vi "Generate write queue item.vi"(8 "error in (no error)":errorcluster, 10 "Request ID":u64, 11 "ICallRequest":refnum<class "ICallRequest.lvclass">) -> (0 "error out":errorcluster, 3 "Write queue item":T1)   [LabVIEW 2020, in "wamplv.lvlib" / "ICallRequest.lvclass"]
uses:
  ICallRequest.lvclass
  WAMP Client/Private/TypeDef/Write queue item.ctl
  TypeDefs/Transport type.ctl
  wamplv.lvlib
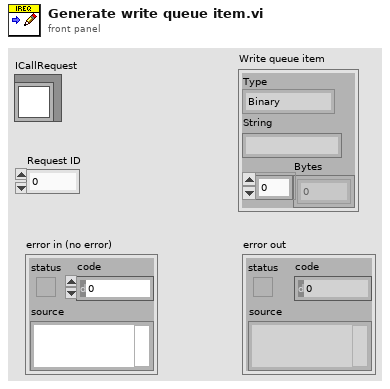
[diagram p1: front panel]
types:
  T1 = typedef "wamplv.lvlib/Write queue item.ctl" = cluster{"Type":T2, "String":string, "Bytes":u8[]}
  T2 = typedef "wamplv.lvlib/Transport type.ctl" = enum16{"Binary", "Text"}
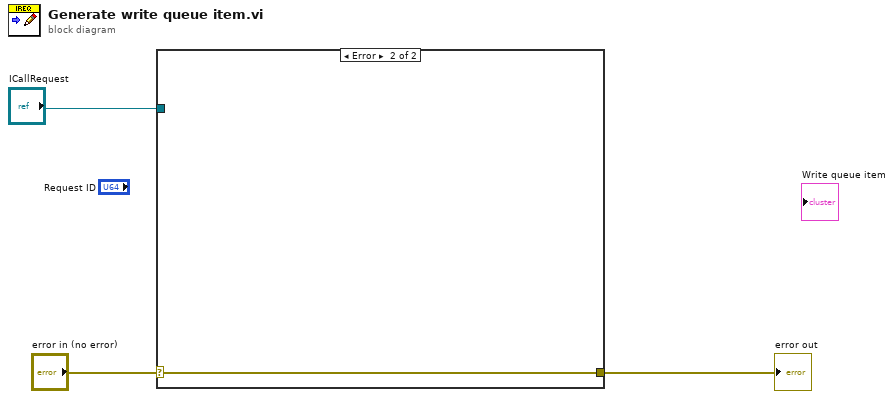
[diagram p0: block diagram]
diagram:
  n1 = case shown="Error" "error in (no error)" {
    selector: "error in (no error)" -> [w4 w5]
    tunnel: [w4 w5] -> w2
    tunnel: "ICallRequest" -> [_ _]
    frame No Error {
      # "Wire the error cluster across even in the \"No Error\"\ncase so that warnings get propagated."
    }
    frame Error {
    }
  }
  "error out" <- w2
